vi "Ternary operator.vi"() -> ()   [LabVIEW 2019]
panel:
  out "Result":string
  in  "Var2":u8
  in  "Var1":u8
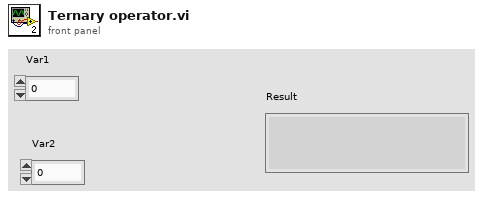
[diagram p1: front panel]
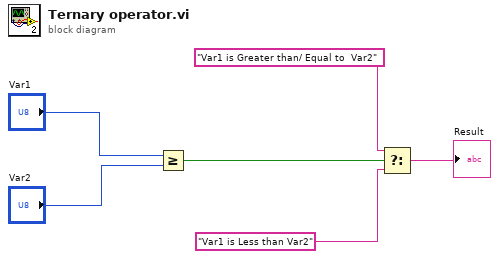
[diagram p0: block diagram]
diagram:
  n1 = Greater Or Equal?(x="Var1", y="Var2") -> (x >= y?=w1:bool)
  n2 = Select(t="Var1 is Greater than/ Equal to  Var2", s=w1, f="Var1 is Less than Var2") -> (s? t:f=→"Result":string)
